vi "MoveCursor.vi"(8 "error in (no error)":errorcluster, 9 "Engine in":refnum<class "Engine.lvclass">, 11 "Highscore in":refnum<class "HighscoreDialog.lvclass">) -> (0 "error out":errorcluster, 1 "Engine out":refnum<class "Engine.lvclass">, 3 "Highscore out":refnum<class "HighscoreDialog.lvclass">)   [LabVIEW 2019, in "RT_Game.lvlib" / "HighscoreDialog.lvclass"]
uses:
  HighscoreDialog.lvclass
  Engine/Engine.lvclass
  HighscoreDialog.lvclass/HighscoreDialog.ctl
  Engine/Engine.lvclass/Engine.ctl
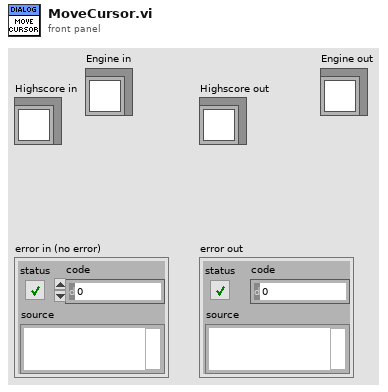
[diagram p1: front panel]
types:
  T1 = typedef "RT_Game.lvlib/Engine.lvclass/Controls.ctl" = cluster{"Controls_1":T2, "Controls_2":cluster{"DirectionX":i8, "DirectionY":i8, "Button1":bool, "Button2":bool}, "SystemButton":bool}
  T2 = typedef "RT_Game.lvlib/Engine.lvclass/ControlPlayer.ctl" = cluster{"DirectionX":i8, "DirectionY":i8, "Button1":bool, "Button2":bool}
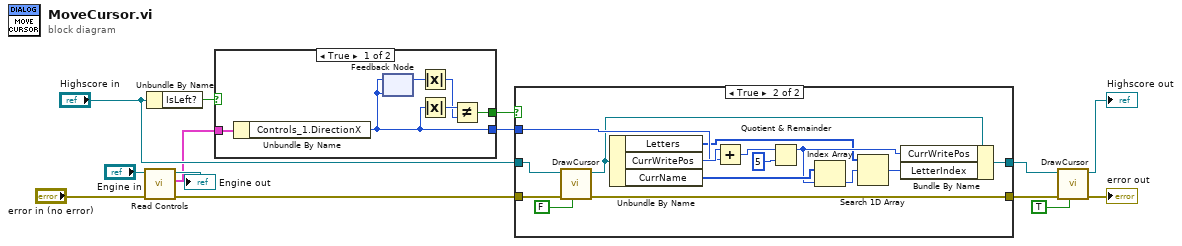
[diagram p0: block diagram]
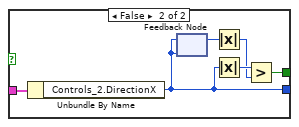
[diagram p3: hidden frame]
diagram:
  n1 = call "Read Controls.vi"("error in (no error)"="error in (no error)", "Engine in"="Engine in") -> ("error out"=w4:errorcluster, "Controls"=w1:T1, "Engine out"=→"Engine out":refnum<class "Engine.lvclass">)  [unwired: 7 in]
  n2 = Unbundle By Name("Highscore in") -> ("IsLeft?"=w13:bool)
  n3 = case shown="True" w13 {
    tunnel: w1 -> [w20 w26]
    tunnel: [w19 w23] -> w10
    tunnel: [w17 w24] -> w11
    frame True {
      n4 = Unbundle By Name(w20) -> ("Controls_1.DirectionX"=w19:i8)
      n5 = feedback-in #1(w19) -> ()
      n6 = feedback #1(w19) -> (w18:i8)
      n7 = Absolute Value(x=w18) -> (abs(x)=w15:i8)
      n8 = Absolute Value(x=w19) -> (abs(x)=w16:i8)
      n9 = Not Equal?(x=w16, y=w15) -> (x != y?=w17:bool)
    }
    frame False {
      n10 = Unbundle By Name(w26) -> ("Controls_2.DirectionX"=w23:i8)
      n11 = feedback #2(w23) -> (w25:i8)
      n12 = feedback-in #2(w23) -> ()
      n13 = Absolute Value(x=w25) -> (abs(x)=w21:i8)
      n14 = Absolute Value(x=w23) -> (abs(x)=w22:i8)
      n15 = Greater?(x=w22, y=w21) -> (0:w24:bool)
    }
  }
  n16 = case shown="True" w11 {
    tunnel: [w28 w33] -> w6
    tunnel: "Highscore in" -> [w28 w31]
    tunnel: w10 -> [_ w41]
    tunnel: w4 -> [w27 w34]
    tunnel: [w27 w32] -> w7
    frame False {
    }
    frame True {
      n17 = call "DrawCursor.vi"("Visible?"=FALSE, "error in (no error)"=w34, "Highscore in"=w31) -> ("error out"=w32:errorcluster, "Highscore out"=w30:refnum<class "HighscoreDialog.lvclass">)  [unwired: 7 in]
      n18 = Unbundle By Name(w30) -> ("Letters"=w37:u8[], "CurrWritePos"=w43:i16, "CurrName"=w39:u8[])
      n19 = Add(x=w43, y=w41) -> (x+y=w42:i16)
      n20 = Quotient & Remainder(x=w42, y=i16 5 ("x")) -> (x-y*floor(x/y)=w38:i16)  [unwired: 1 out]
      n21 = Index Array(array=w39, index=w38) -> (element=w36:u8)
      n22 = Search 1D Array(1D array=w37, element=w36) -> (index of element=w35:i32)  [unwired: 1 in]
      n23 = Bundle By Name(cluster=w30, "CurrWritePos"=w38, "LetterIndex"=w35) -> (w33:refnum<class "HighscoreDialog.lvclass">)
    }
  }
  n24 = call "DrawCursor.vi"("Visible?"=TRUE, "error in (no error)"=w7, "Highscore in"=w6) -> ("error out"=→"error out":errorcluster, "Highscore out"=→"Highscore out":refnum<class "HighscoreDialog.lvclass">)  [unwired: 7 in]
